vi "Read Msg Ref.vi"(11 "Event Transport in":refnum<class "Event Transport.lvclass">) -> (2 "Msg Ref":refnum<event-registration>)   [LabVIEW 2025, in "jettl.lvlib" / "Transport.lvlib" / "Event.lvlib" / "Event Transport.lvclass"]
uses:
  Event Transport.lvclass
  Msg/Msg.lvclass
  Event Transport.lvclass/Event Transport.ctl
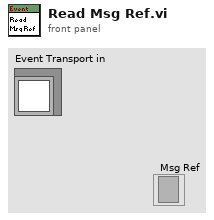
[diagram p1: front panel]
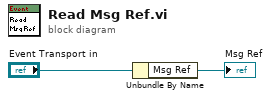
[diagram p0: block diagram]
diagram:
  n1 = Unbundle By Name("Event Transport in") -> ("Msg Ref"=→"Msg Ref":refnum<event-registration>)
